vi "State_Checker.vi"(0 "Linked index":i32[](array[numeric]), 1 "Index":i32, 2 "Actions":i32[][](array[numeric]), 4 "Current time":timestamp, 6 "Time of last action":timestamp[](array[timestamp]), 8 "Action count in":i32[](array[numeric]), 12 "Immediate actions in":bool[](array[boolean])) -> (23 "State Ready?":bool, 26 "Time of next out":timestamp)   [LabVIEW 2025]
uses:
  TypeDef_State_Action_Columns.ctl
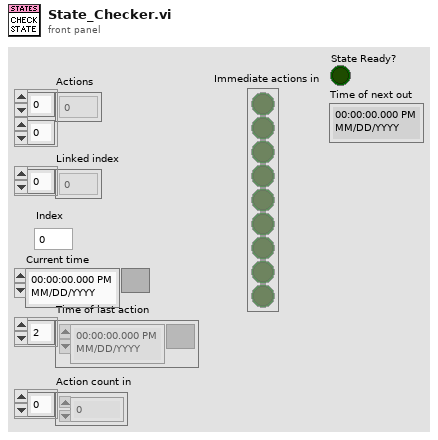
[diagram p1: front panel]
types:
  T1 = typedef "TypeDef_State_Action_Columns.ctl" = enum16{"Action_num", "trigger", "fequency", "offset", "initial state", "mode", "order", "link", "description"}
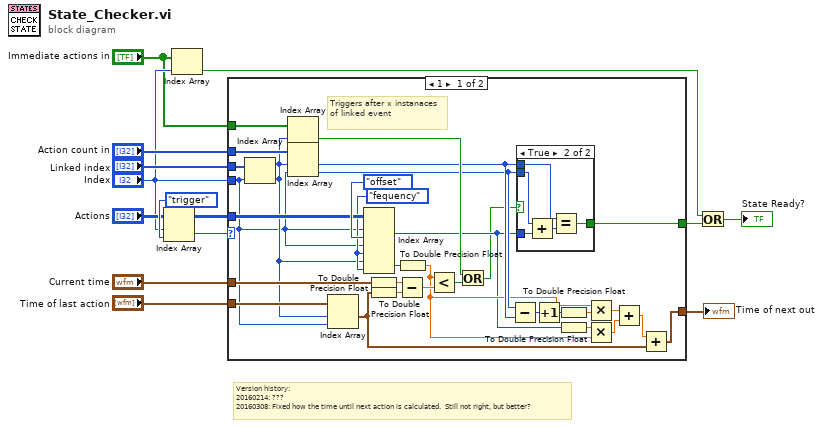
[diagram p0: block diagram]
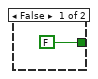
[diagram p2: hidden frame]
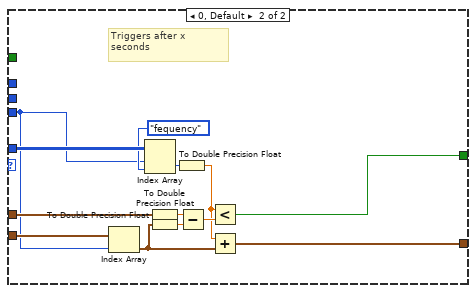
[diagram p3: hidden frame]
diagram:
  # "Version history:\n20160214: ???\n20160308: Fixed how the time until next action is calculated.  Still not right, but better?"
  n1 = Index Array(array="Actions", index (row)="Index", index (col)=TypeDef_State_Action_Columns."trigger" ("Enum")) -> (element=w1:i32)
  n2 = Index Array(array="Immediate actions in", index="Index") -> (element=w5:bool)
  n3 = case shown="1" w1 {
    tunnel: "Actions" -> [w38 w60]
    tunnel: "Current time" -> [w37 w59]
    tunnel: "Time of last action" -> [w35 w55]
    tunnel: [w16 w57] -> w13
    tunnel: "Action count in" -> [w44 _]
    tunnel: "Linked index" -> [w43 _]
    tunnel: [w29 w56] -> w6
    tunnel: "Index" -> [w30 w53]
    tunnel: "Immediate actions in" -> [w34 _]
    frame 1 {
      w36 = TypeDef_State_Action_Columns."fequency" ("Enum")
      # "Triggers after x instanaces of linked event"
      n4 = Index Array(array=w43, index=w30) -> (element=w33:i32)
      n5 = Index Array(array=w34, index=w33) -> (element=w31:bool)
      n6 = Index Array(array=w44, index #1=w33, index #2=w30) -> (element #1=w28:i32, element #2=w27:i32)
      n7 = Index Array(array=w35, index #1=w33, index #2=w30) -> (element #1=w26:timestamp)  [unwired: 1 out]
      n8 = Index Array(array=w38, index (row) #1=w30, index (col) #1=TypeDef_State_Action_Columns."offset" ("Enum"), index (row) #2=w30, index (col) #2=w36, index (row) #3=w33, index (col) #3=w36) -> (element #1=w18:i32, element #3=w25:i32)  [unwired: 1 out]
      n9 = To Double Precision Float(number=w37) -> (double precision float=w40:dbl)
      n10 = To Double Precision Float(number=w26) -> (double precision float=w39:dbl)
      n11 = Subtract(x=w40, y=w39) -> (x-y=w41:dbl)
      n12 = To Double Precision Float(number=w25) -> (double precision float=w23:dbl)
      n13 = Less?(x=w23, y=w41) -> (x < y?=w32:bool)
      n14 = Or(x=w31, y=w32) -> (x .or. y?=w17:bool)
      n15 = Subtract(x=w27, y=w28) -> (x-y=w15:i32)
      n16 = case shown="True" w17 {
        tunnel: [FALSE w49] -> w16
        tunnel: w28 -> [_ w46]
        tunnel: w27 -> [_ w47]
        tunnel: w18 -> [_ w48]
        frame False {
        }
        frame True {
          n17 = Add(x=w47, y=w48) -> (x+y=w50:i32)
          n18 = Equal?(x=w46, y=w50) -> (x = y?=w49:bool)
        }
      }
      n19 = Increment(x=w15) -> (x+1=w14:i32)
      n20 = To Double Precision Float(number=w14) -> (double precision float=w24:dbl)
      n21 = To Double Precision Float(number=w18) -> (double precision float=w19:dbl)
      n22 = Multiply(x=w23, y=w24) -> (x*y=w22:dbl)
      n23 = Multiply(x=w19, y=w23) -> (x*y=w21:dbl)
      n24 = Add(x=w22, y=w21) -> (x+y=w20:dbl)
      n25 = Add(x=w20, y=w26) -> (x+y=w29:timestamp)
    }
    frame 0, Default {
      # "Triggers after x seconds"
      n26 = Index Array(array=w55, index=w53) -> (element=w54:timestamp)
      n27 = Index Array(array=w60, index (row)=w53, index (col)=TypeDef_State_Action_Columns."fequency" ("Enum")) -> (element=w52:i32)
      n28 = To Double Precision Float(number=w59) -> (double precision float=w62:dbl)
      n29 = To Double Precision Float(number=w54) -> (double precision float=w61:dbl)
      n30 = To Double Precision Float(number=w52) -> (double precision float=w51:dbl)
      n31 = Subtract(x=w62, y=w61) -> (x-y=w63:dbl)
      n32 = Less?(x=w51, y=w63) -> (x < y?=w57:bool)
      n33 = Add(x=w51, y=w54) -> (x+y=w56:timestamp)
    }
  }
  "Time of next out" <- w6
  n34 = Or(x=w5, y=w13) -> (x .or. y?=→"State Ready?":bool)
